vi "TA_Generate_DelayTime_LoadfromFile.vi"(11 "File Path":path=path "/Users/tm/Desktop/fs-TA/Data/demo_fsta.dat") -> (2 "Number (Delay Time)":i32, 3 "Generated Delay Time (ps)":dbl[](array[numeric]))   [LabVIEW 2025]
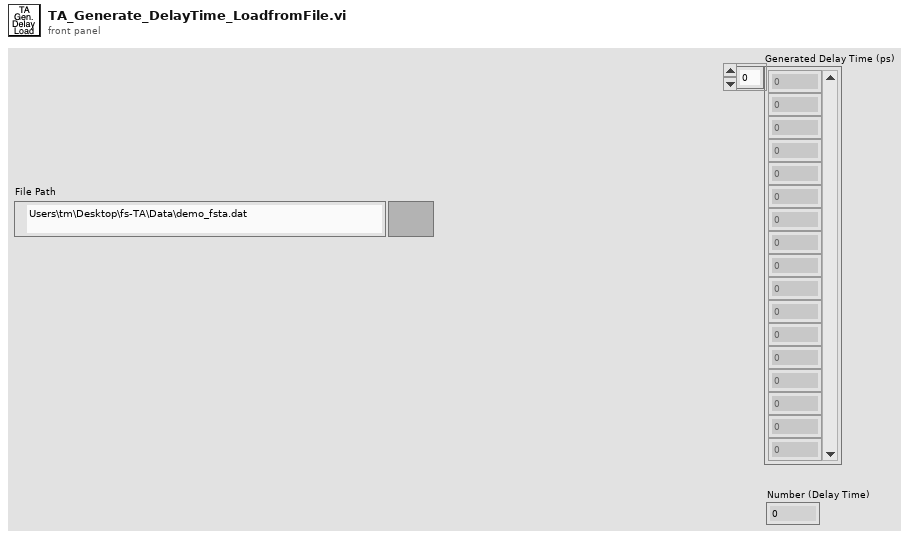
[diagram p1: front panel]
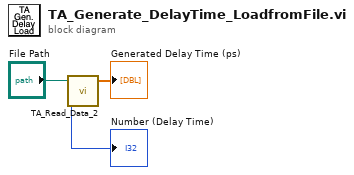
[diagram p0: block diagram]
diagram:
  n1 = call "TA_Read_Data_2.vi"("File Path"="File Path") -> ("size(delay time)"=→"Number (Delay Time)":i32, "delay time (ps)"=→"Generated Delay Time (ps)":dbl[])  [unwired: 1 in, 4 out]
